vi "Task Type.vi"(11 "DaqControl in":refnum<class "DaqControl.lvclass">) -> (2 "Task Type":string)   [LabVIEW 2020, in "VolatusDaq.lvlib" / "DaqControl.lvclass"]
uses:
  DaqControl.lvclass
  DaqControl.lvclass/DaqControl.ctl
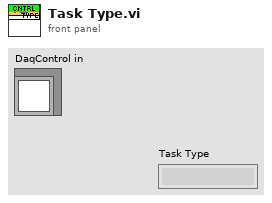
[diagram p1: front panel]
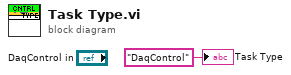
[diagram p0: block diagram]
diagram:
  "Task Type" <- "DaqControl" ("Task Type")
